vi "Limelight_Differential.vi"() -> (0 "TargetValid":bool, 2 "SteerCommand":dbl(knob)=nan scale=-1.0..1.0, 3 "DriveCommand":dbl(knob)=-0.0 scale=-1.0..1.0)   [LabVIEW 2020]
uses:
  <vilib>/Rock Robotics/Network Tables/NT Read Number.vi
  Framework/Robot Global Data.vi
panel:
  out "MaxDrive":dbl(slide)=0.6824817518248175 min=0.0 max=1.0 step=0.01 scale=0.0..1.0
  out "DriveK":dbl(slide)=0.26277372262773724 min=0.0 max=1.0 step=0.05 scale=0.0..1.0
  out "Limelight Goal Area":dbl(slide)=14.8723 min=0.1 max=25.0 step=0.25 scale=0.0..25.0
  out "AimDeadband":dbl min=0.0 max=10.0 step=0.25
  out "MinSteerCommand":dbl(slide)=0.2717391304347826 min=0.0 max=0.5 step=0.05 scale=0.0..0.5
  out "SteeringK":dbl(slide)=0.025362318840579712 min=0.0 max=0.25 step=0.01 scale=0.0..0.25
  # "0.0253623"
  # "0.271739"
  # "14.8723"
  # "0.262774"
  # "0.682482"
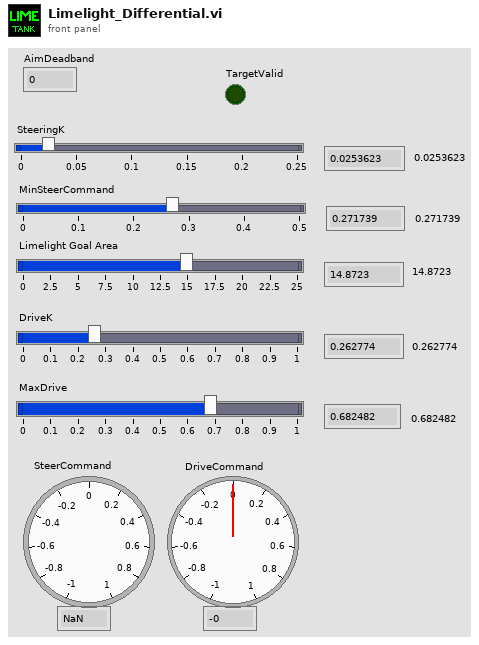
[diagram p1: front panel]
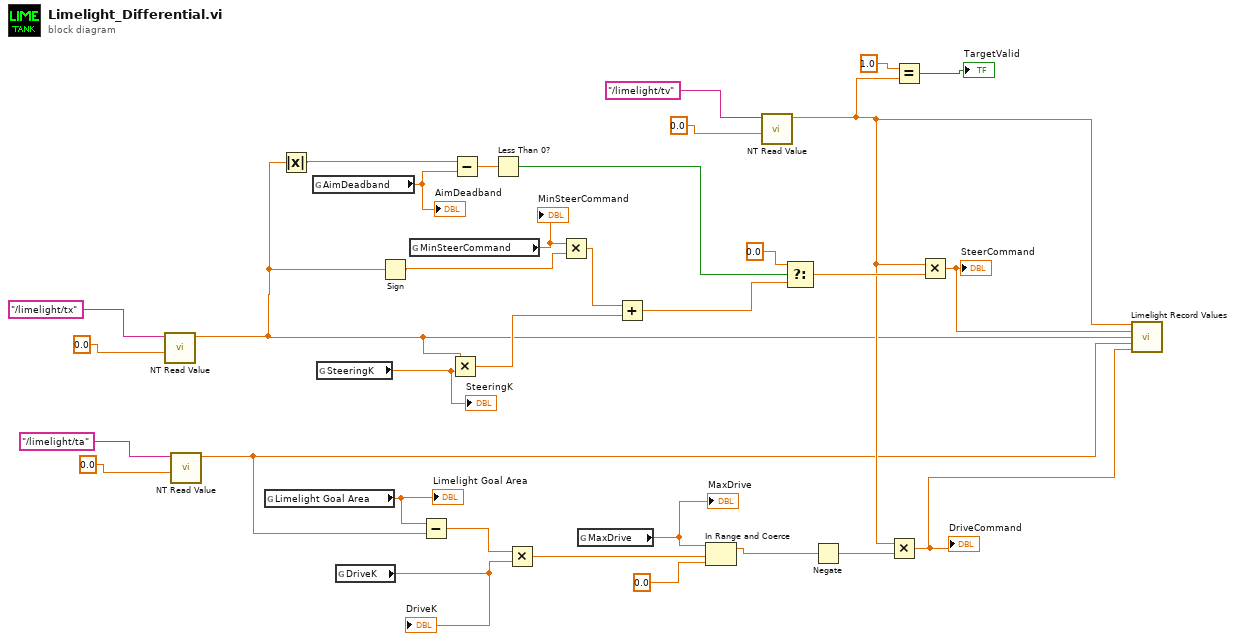
[diagram p0: block diagram]
diagram:
  n1 = call-poly <vilib>:"NT Read Value.vi"("Default Value"=0.0, "Name"="/limelight/tx") -> ("Numeric"=w3:dbl)  [unwired: 8 in, 1 out]
  n2 = call-poly <vilib>:"NT Read Value.vi"("Default Value"=0.0, "Name"="/limelight/ta") -> ("Numeric"=w2:dbl)  [unwired: 8 in, 1 out]
  n3 = global read "Robot Global Data.vi" "Limelight Goal Area"() -> (w8:dbl)
  "Limelight Goal Area" <- w8
  n4 = Absolute Value(x=w3) -> (abs(x)=w30:dbl)
  n5 = global read "Robot Global Data.vi" "AimDeadband"() -> (w11:dbl)
  "AimDeadband" <- w11
  n6 = global read "Robot Global Data.vi" "SteeringK"() -> (w9:dbl)
  "SteeringK" <- w9
  n7 = global read "Robot Global Data.vi" "DriveK"() -> (w6:dbl)
  "DriveK" <- w6
  n8 = Sign(1:w3) -> (0:w20:dbl)
  n9 = global read "Robot Global Data.vi" "MinSteerCommand"() -> (w10:dbl)
  "MinSteerCommand" <- w10
  n10 = Subtract(x=w8, y=w2) -> (x-y=w19:dbl)
  n11 = Multiply(x=w3, y=w9) -> (x*y=w28:dbl)
  n12 = Subtract(x=w30, y=w11) -> (x-y=w31:dbl)
  n13 = Less Than 0?(x=w31) -> (x < 0?=w32:bool)
  n14 = Multiply(x=w19, y=w6) -> (x*y=w18:dbl)
  n15 = Multiply(x=w10, y=w20) -> (x*y=w29:dbl)
  n16 = global read "Robot Global Data.vi" "MaxDrive"() -> (w7:dbl)
  "MaxDrive" <- w7
  n17 = Add(x=w29, y=w28) -> (x+y=w14:dbl)
  n18 = In Range and Coerce(upper limit=w7, x=w18, lower limit=0.0) -> (coerced(x)=w16:dbl)  [unwired: 1 out]
  n19 = call-poly <vilib>:"NT Read Value.vi"("Default Value"=0.0, "Name"="/limelight/tv") -> ("Numeric"=w5:dbl)  [unwired: 8 in, 1 out]
  n20 = Select(t=0.0, s=w32, f=w14) -> (s? t:f=w21:dbl)
  n21 = Negate(x=w16) -> (-x=w15:dbl)
  n22 = Multiply(x=w5, y=w15) -> (x*y=w1:dbl)
  "DriveCommand" <- w1
  n23 = Equal?(x=1.0, y=w5) -> (x = y?=→"TargetValid":bool)
  n24 = Multiply(x=w5, y=w21) -> (x*y=w4:dbl)
  "SteerCommand" <- w4
  n25 = call "Limelight Record Values.vi"("tv"=w5, "Steer"=w4, "tx"=w3, "ta"=w2, "Drive"=w1) -> ()  [unwired: 11 in]
